vi "Get MD5 For File.vi"(8 "error in":errorcluster, 11 "path":path) -> (0 "error out":errorcluster, 1 "MD5":string)   [LabVIEW 2024]
uses:
  NationalInstruments.VeriStand.Internal
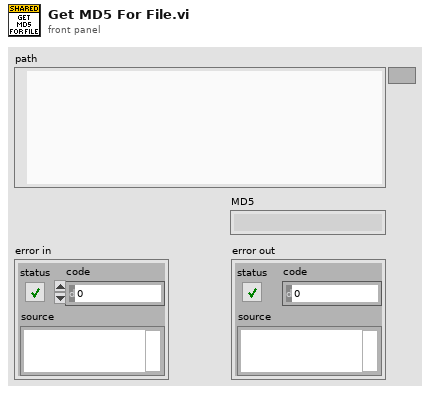
[diagram p1: front panel]
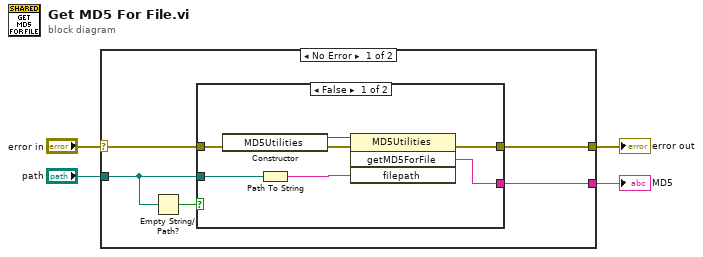
[diagram p0: block diagram]
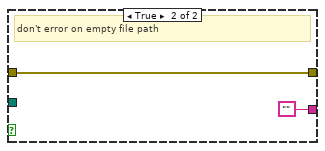
[diagram p2: hidden frame]
diagram:
  n1 = case shown="No Error" "error in" {
    selector: "error in" -> [w9 w19]
    tunnel: [w8 w19] -> w2
    tunnel: "path" -> [w5 _]
    tunnel: [w7 _] -> w1
    frame No Error {
      n2 = Empty String/Path?(string/path=w5) -> (empty?=w6:bool)
      n3 = case shown="False" w6 {
        tunnel: w9 -> [w13 w18]
        tunnel: w5 -> [w12 _]
        tunnel: [w11 w18] -> w8
        tunnel: [w10 ""] -> w7
        frame False {
          n4 = constructor class="MD5Utilities"(error in=w13) -> (reference out=w14:refnum<k24>, error out=w15:errorcluster)  [unwired: 2 in, 1 out]
          n5 = Path To String(path=w12) -> (string=w16:string)
          n6 = invoke class="MD5Utilities" method="getMD5ForFile"(reference=w14, error in=w15, "filepath"=w16) -> (error out=w11:errorcluster, "getMD5ForFile"=w10:string)  [unwired: 1 in, 2 out]
        }
        frame True {
          # "don't error on empty file path"
        }
      }
    }
    frame Error {
    }
  }
  "error out" <- w2
  "MD5" <- w1
